vi "V7310.Stop.vi"(6 "timeout ms (5000)":i32=5000, 8 "error in":errorcluster, 11 "Connection in":refnum<k5>) -> (0 "error out":errorcluster, 3 "Connection out":refnum<k5>)   [LabVIEW 2016]
uses:
  LowLevel/V7310.Commands.ctl
panel:
  out "Data out":string
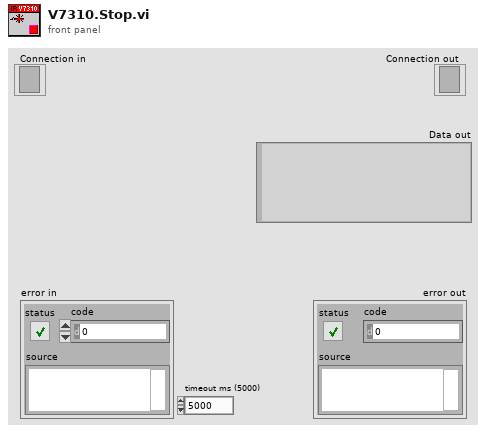
[diagram p1: front panel]
types:
  T1 = typedef "V7310.Commands.ctl" = enum16{"Start", "Stop", "GetStatus", "GetVarNames", "GetJobNames", "SetJob", "GetJob", "SetVars", "GetVars", "SetLayoutPosition", "SetRotation", "GetMessageID", "GetMessages", "ConfirmMessages", "DeleteMessages", "SetRTC", "GetRTC", "SetVarPosition", "SetIntensity", "GetIntensity", "SetStartTriggerDelay", "GetStartTriggerDelay", "SetStopTriggerDelay", "GetStopTriggerDelay", "SetConsecutiveTriggerDelay", "GetConsecutiveTriggerDelay", "SetMarkSpeed", "GetMarkSpeed"}
  T2 = typedef "V7310.ErrorLevels.ctl" = enum16{"OK", "Warning", "Error"}
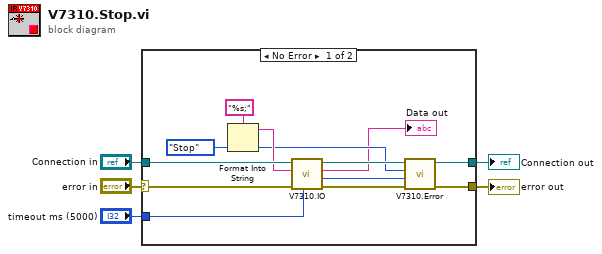
[diagram p0: block diagram]
diagram:
  n1 = case shown="No Error" "error in" {
    selector: "error in" -> [w14 w17]
    tunnel: "Connection in" -> [w15 w18]
    tunnel: [w16 w18] -> w4
    tunnel: "timeout ms (5000)" -> [w13 _]
    tunnel: [w7 w17] -> w1
    frame No Error {
      w10 = V7310.Commands."Stop" ("Cmd")
      n2 = Format Into String(format string="%s;", w10) -> (resulting string=w11:string)  [unwired: 2 in, 1 out]
      n3 = call "V7310.IO.vi"("timeout ms (5000)"=w13, "error in"=w14, "Data in"=w11, "Connection in"=w15) -> ("error out"=w8:errorcluster, "Error Level"=w9:T2, "Data out"=→"Data out":string, "Connection out"=w16:refnum<k5>)  [unwired: 4 in]
      n4 = call "V7310.Error.vi"("error in"=w8, "Error Level"=w9, "Cmd"=w10) -> ("error out"=w7:errorcluster)  [unwired: 8 in]
    }
    frame Error {
    }
  }
  "Connection out" <- w4
  "error out" <- w1
